vi "PNA_MAIN_RF_POWER.vi"(0 "Session In":refnum<visa-resource-name>="TCPIP0::169.254.70.180::inst0::INSTR", 5 "error in":errorcluster {"code" format="%.0x"}, 7 "LEVEL(DBM)":dbl, 8 "Timeout":u32=5000, 10 "RO(T)":bool, 11 "CH":i32=1, 13 "Source":i32=1) -> (12 "level(dbm)":dbl, 14 "Session Out":refnum<visa-resource-name>="TCPIP0::169.254.70.180::inst0::INSTR", 19 "error out":errorcluster {"code" format="%.0x"})   [LabVIEW 2018]
doc: "Applicable Models: All\n\n(Read-Write) Sets the RF power output level.\n \nParameters\n \n \n<cnum>\n Any existing channel number. If unspecified, value is set to 1\n \n<port>\n Source port number of the VNA. If unspecified, value is set to 1. To make settings for ports that are not simple numbers, use the [src] argument.\n \n<num>\n Source power in dBm.\n\nNote: The range of settable power values depends on the VNA model and if source attenuators are installed. To determine the range of values, perform a query using MAX, then MIN, as an argument. (SOUR:POW:ATT:AUTO must be set to ON) Example: SOURce:POWer? Max\n\nActual achievable leveled power depends on frequency.\n \n[src]\n String. (NOT case sensitive). Source port. Optional. Use SOUR:CAT? to return a list of valid port names.\n\nWhile this argument can be used to make settings for ALL ports, it is designed to access ports such as an external source, true mode balanced port, or one of the Source 2 outputs on the 2-port 2-source PNA-X model such as \"Port 1 Src2\". Otherwise, the <port> argument performs the same function. If both arguments are specified, [src] takes priority"
panel:
  out "Rd String":string="sour1:pow1:LEV:IMM:AMPL?"
  out "Wr String":string="sour1:pow1:LEV:IMM:AMPL 0.000000\n"
  # "Instrument Address"
  # "Select Source"
  # "Conditions"
  # "Is Read Only (T)"
  # "Channel"
  # "Source"
  # "Inst Timeout(ms)"
  # "Set Level"
  # "Level (dBm)"
  # "Read (dBm)"
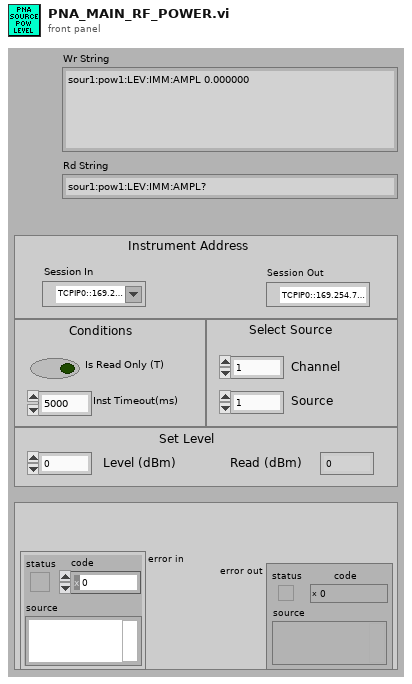
[diagram p1: front panel]
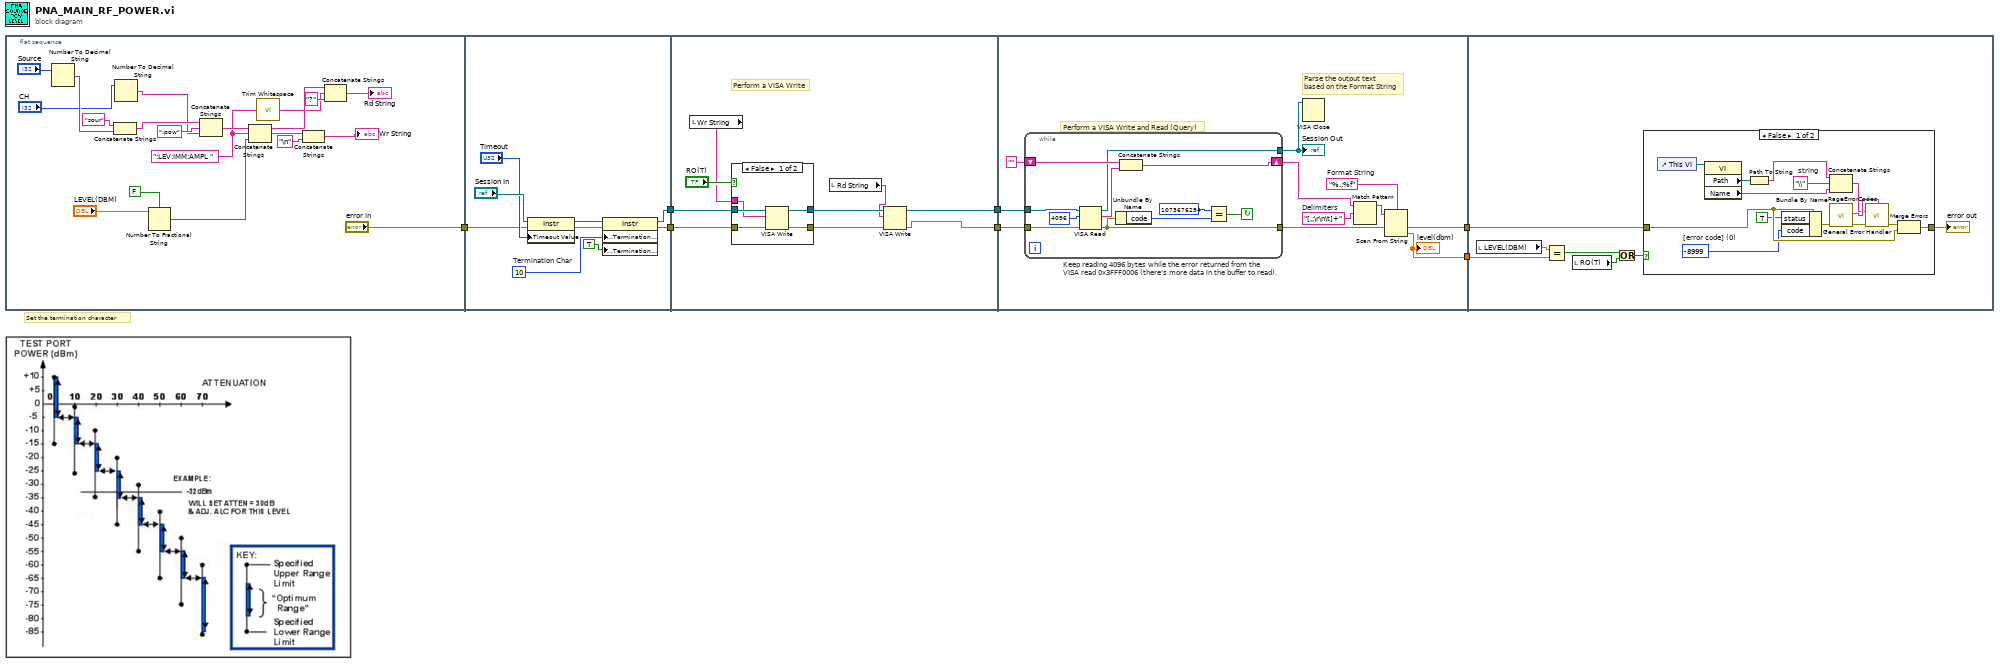
[diagram p0: block diagram]
diagram:
  # "Set the termination character"
  n1 = flat-sequence {
    tunnel: ["error in"] -> w1
    tunnel: [w29] -> w7
    tunnel: [w28] -> w6
    tunnel: w1 -> [w27]
    tunnel: w7 -> [w43]
    tunnel: w6 -> [w44]
    tunnel: [w37] -> w5
    tunnel: [w36] -> w4
    tunnel: w5 -> [w54]
    tunnel: w4 -> [w56]
    tunnel: [w53] -> w3
    tunnel: [w52] -> w2
    tunnel: w3 -> [w75]
    tunnel: w2 -> [w74]
    frame #0 {
      w11 = ":LEV:IMM:AMPL " ("staticText")
      n2 = Number To Decimal String(number="Source") -> (decimal integer string=w18:string)  [unwired: 1 out]
      n3 = Concatenate Strings("sour" ("staticText"), w18) -> (w23:string)
      n4 = Number To Decimal String(number="CH") -> (decimal integer string=w17:string)  [unwired: 1 out]
      n5 = Number To Fractional String(use system decimal point (T)=FALSE, number="LEVEL(DBM)") -> (F-format string=w21:string)  [unwired: 2 in]
      n6 = Concatenate Strings(w23, ":pow" ("staticText"), w17) -> (w12:string)
      n7 = Concatenate Strings(w12, w11, w21) -> (w20:string)
      n8 = call <vilib>:"Trim Whitespace.vi"("string"=w11) -> ("trimmed string"=w8:string)  [unwired: 1 in]
      n9 = Concatenate Strings(w20, "\n" ("StaticText")) -> (→"Wr String":string)
      n10 = Concatenate Strings(w12, w8, "?" ("string")) -> (→"Rd String":string)
    }
    frame #1 {
      w32 = u8 10  # Termination Char
      n11 = property class="Instr"(reference="Session In", error in=w27, "General Settings:Timeout Value"="Timeout") -> (reference out=w34:refnum<visa-resource-name>, error out=w33:errorcluster)
      n12 = property class="Instr"(reference=w34, error in=w33, "Message Based Settings:Termination Character"=w32, "Message Based Settings:Termination Character Enable"=TRUE ("enable")) -> (reference out=w29:refnum<visa-resource-name>, error out=w28:errorcluster)
    }
    frame #2 {
      # "Perform a VISA Write"
      n13 = local read "Wr String"() -> (w38:string)
      n14 = case shown="False" "RO(T)" {
        tunnel: w44 -> [w49 w50]
        tunnel: [w48 w50] -> w40
        tunnel: w38 -> [w45 _]
        tunnel: w43 -> [w47 w51]
        tunnel: [w46 w51] -> w41
        frame False {
          n15 = VISA Write(VISA resource name=w47, write buffer=w45, error in (no error)=w49) -> (VISA resource name out=w46:refnum<visa-resource-name>, error out=w48:errorcluster)  [unwired: 1 out]
        }
        frame True {
        }
      }
      n16 = local read "Rd String"() -> (w39:string)
      n17 = VISA Write(VISA resource name=w41, write buffer=w39, error in (no error)=w40) -> (VISA resource name out=w36:refnum<visa-resource-name>, error out=w37:errorcluster)  [unwired: 1 out]
    }
    frame #3 {
      w58 = "[,;\r\n\t]+"  # Delimiters
      w57 = "%.;%f"  # Format String
      # "Parse the output text based on the Format String"
      # "Perform a VISA Write and Read (Query)"
      # "Keep reading 4096 bytes while the error returned from the\nVISA read 0x3FFF0006 (there's more data in the buffer to read)."
      n18 = while {
        tunnel: w56 -> [w70]
        shift-right: [w64] -> w60
        shift-left: "" -> [w69]
        tunnel: w54 -> [w67]
        tunnel: [w66] -> w59
        tunnel: [w63] -> w62
        stop <- w65 continue-if-true
        n19 = VISA Read(VISA resource name=w70, byte count=u32 4096 ("byte count (0)"), error in (no error)=w67) -> (VISA resource name out=w63:refnum<visa-resource-name>, read buffer=w68:string, error out=w66:errorcluster)  [unwired: 1 out]
        n20 = Unbundle By Name(w66) -> ("code"=w72:i32)
        n21 = Concatenate Strings(w69, w68) -> (w64:string)
        n22 = Equal?(x=1073676294, y=w72) -> (x = y?=w65:bool)
      }
      "Session Out" <- w62
      n23 = VISA Close(VISA resource name=w62) -> ()  [unwired: 1 in, 1 out]
      n24 = Match Pattern(string=w60, regular expression=w58) -> (before substring=w61:string)  [unwired: 1 in, 3 out]
      n25 = Scan From String(format string=w57, input string=w61, error in=w59) -> (error out=w53:errorcluster, output 1=w52:dbl)  [unwired: 2 in, 2 out]
      "level(dbm)" <- w52
    }
    frame #4 {
      n26 = local read "LEVEL(DBM)"() -> (w76:dbl)
      n27 = Equal?(x=w76, y=w74) -> (x = y?=w78:bool)
      n28 = local read "RO(T)"() -> (w79:bool)
      n29 = Or(x=w78, y=w79) -> (x .or. y?=w80:bool)
      n30 = case shown="False" w80 {
        tunnel: w75 -> [w84 w95]
        tunnel: [w85 w95] -> w77
        frame False {
          w87 = "\\"  # string
          w82 = -8999  # [error code] (0)
          n31 = control-ref of="This VI"() -> (w92:refnum<vi>)
          n32 = property class="VI"(reference=w92) -> ("Path"=w90:path, "Name"=w88:string)  [unwired: 1 in, 2 out]
          n33 = Path To String(path=w90) -> (string=w89:string)
          n34 = Bundle By Name(cluster=w84, "status"=TRUE, "code"=w82) -> (w81:errorcluster)
          n35 = Concatenate Strings(w89, w87, w88) -> (w91:string)
          n36 = call "RageErrorCodes.vi"("error in"=w81) -> ("error out"=w94:errorcluster, "desc ary"=w93:string[])  [unwired: 8 in, 1 out]
          n37 = call <vilib>:"General Error Handler.vi"("[user-defined descriptions]"=w93, "[error source] (\" \")"=w91, "error in (no error)"=w94) -> ("error out"=w86:errorcluster)  [unwired: 8 in, 4 out]
          n38 = Merge Errors(w86, w84) -> (w85:errorcluster)
        }
        frame True {
        }
      }
      "error out" <- w77
    }
  }
